vi "Publish Report.vi"(8 "error in (no error)":errorcluster, 11 "Report in":refnum<class "Report.lvclass">) -> (0 "error out":errorcluster, 3 "Report out":refnum<class "Report.lvclass">)   [LabVIEW 2015, in "Report.lvclass"]
doc: "This VI will write the in-memory report to disk."
uses:
  Report.lvclass
  Report.lvclass/Report.ctl
  Report Information/Report Information.lvclass
  Result/Result.lvclass
  Report Formatters/Base Class/Formatter.lvclass
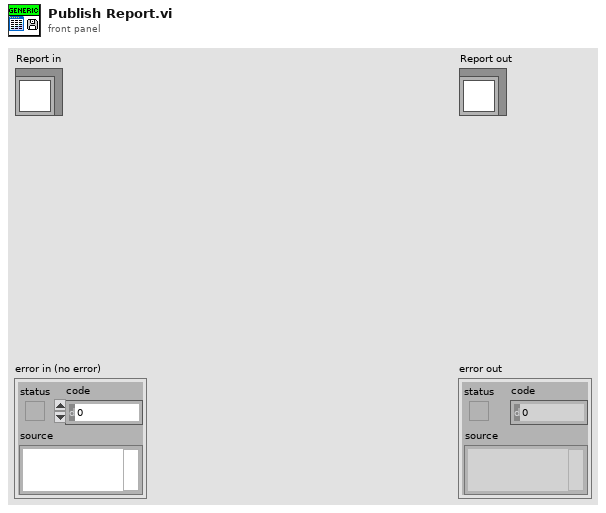
[diagram p1: front panel]
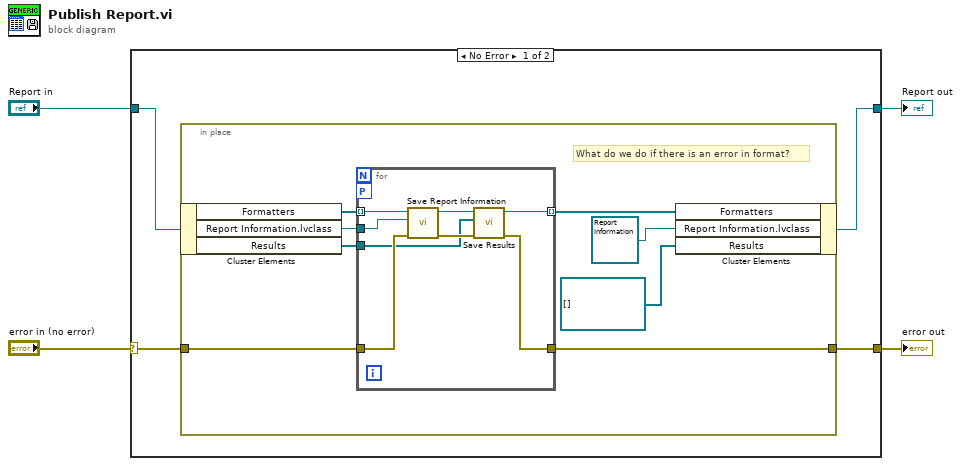
[diagram p0: block diagram]
diagram:
  n1 = case shown="No Error" "error in (no error)" {
    selector: "error in (no error)" -> [w8 w26]
    tunnel: [w7 w26] -> w3
    tunnel: [w5 w25] -> w1
    tunnel: "Report in" -> [w6 w25]
    frame No Error {
      n2 = in-place {
        in-place-border: w8 -> [w16]
        in-place-border: [w15] -> w7
        # "What do we do if there is an error in format?"
        n3 = in-place-cluster #1(w6) -> ("Formatters"=w14:refnum<class "Formatter.lvclass">[], "Report Information.lvclass"=w13:refnum<class "Report Information.lvclass">, "Results"=w12:refnum<class "Result.lvclass">[])
        n4 = for {
          tunnel: w16 -> [w22]
          tunnel: [w19] -> w15
          tunnel: w14 -> [w24] mode=indexing
          tunnel: w13 -> [w23]
          tunnel: w12 -> [w18]
          tunnel: [w17] -> w11 mode=indexing
          workers-P: _ -> [_]
          n5 = call-dynamic "Save Report Information.vi"("error in (no error)"=w22, "Report Information.lvclass"=w23, "Formatter in"=w24) -> ("error out"=w20:errorcluster, "Formatter out"=w21:refnum<class "Formatter.lvclass">)  [unwired: 7 in]
          n6 = call-dynamic "Save Results.vi"("error in (no error)"=w20, "Results"=w18, "Formatter in"=w21) -> ("error out"=w19:errorcluster, "Formatter out"=w17:refnum<class "Formatter.lvclass">)  [unwired: 7 in]
        }
        n7 = in-place-cluster #1("Formatters"=w11, "Report Information.lvclass"=refnum<class "Report Information.lvclass"> refnum, "Results"=refnum<class "Result.lvclass">[] []) -> (w5:refnum<class "Report.lvclass">)
      }
    }
    frame Error {
    }
  }
  "error out" <- w3
  "Report out" <- w1
